vi "Stop.vi"(8 "error in (no error)":errorcluster, 11 "Report Generator In":refnum<class "Report Generator.lvclass">) -> (0 "error out":errorcluster, 3 "Report Generator Out":refnum<class "Report Generator.lvclass">)   [LabVIEW 2020, in "Report Generation.lvlib" / "Report Generator.lvclass"]
uses:
  Report Generator.lvclass
  C:/git/astemes-lunit/source/User Interface/Process/Process.lvclass
  User Interface/Process/Process.lvclass/Process.ctl
  User Interface/Process/Process.lvclass
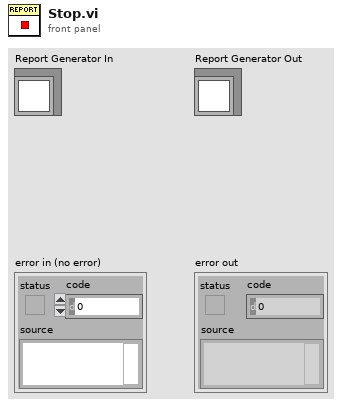
[diagram p1: front panel]
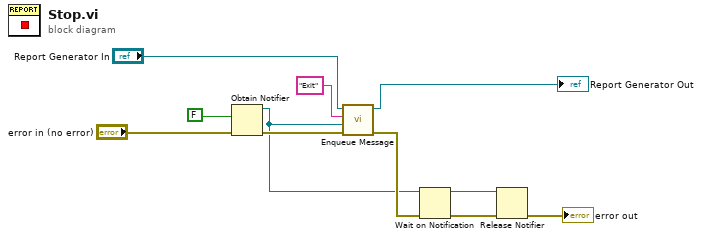
[diagram p0: block diagram]
diagram:
  n1 = Obtain Notifier(notification data type=FALSE, error in (no error)="error in (no error)") -> (notifier out=w3:refnum<notifier>, error out=w6:errorcluster)  [unwired: 2 in, 1 out]
  n2 = call "Enqueue Message.vi"("error in (no error)"=w6, "Message Data"=w3, "Message"="Exit", "Process In"="Report Generator In") -> ("error out"=w8:errorcluster, "Process Out"=→"Report Generator Out":refnum<class "Report Generator.lvclass">)  [unwired: 6 in]
  n3 = Wait on Notification(notifier=w3, error in (no error)=w8) -> (notifier out=w1:refnum<notifier>, error out=w4:errorcluster)  [unwired: 2 in, 2 out]
  n4 = Release Notifier(notifier=w1, error in (no error)=w4) -> (error out=→"error out":errorcluster)  [unwired: 1 in, 2 out]
